vi "OCRListAvialableLangs_Training.vi"(8 "error in (no error)":errorcluster) -> (0 "error out":errorcluster, 3 "Langs":string[](array[string]))   [LabVIEW 2019]
panel:
  out "standard error":string
  out "standard output":string
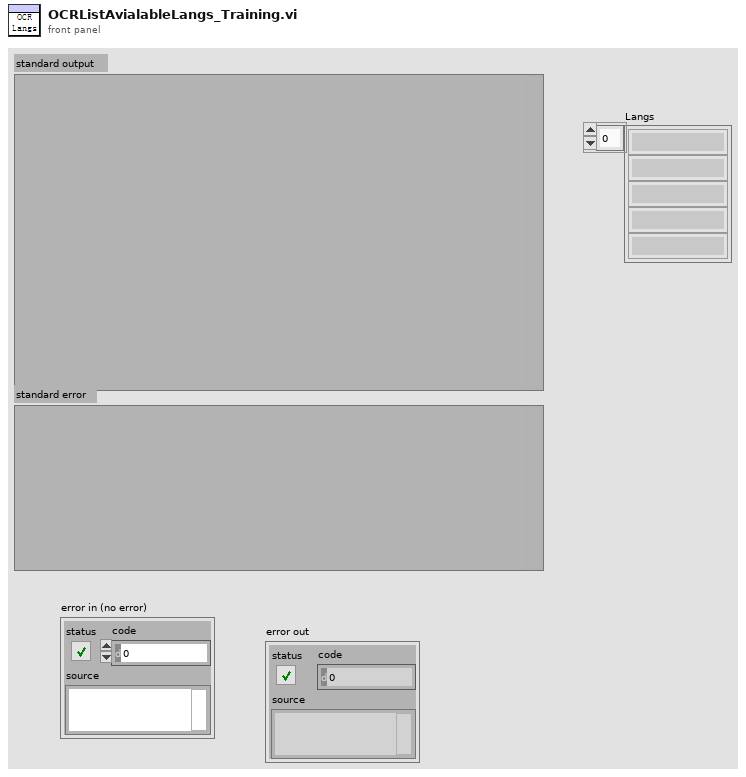
[diagram p1: front panel]
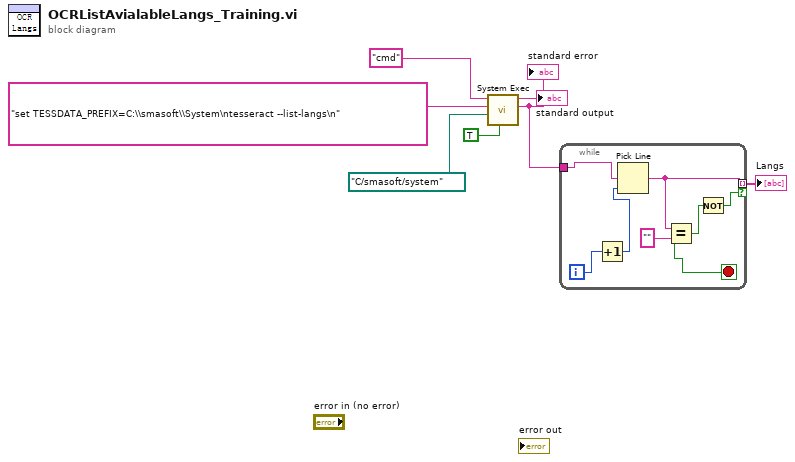
[diagram p0: block diagram]
diagram:
  n1 = call <vilib>:"System Exec.vi"("run minimized? (F)"=TRUE, "working directory"=path "C:/smasoft/system", "standard input"="set TESSDATA_PREFIX=C:\\smasoft\\System\ntesseract --list-langs\n", "command line"="cmd") -> ("standard error"=w2:string, "standard output"=→"standard output":string)  [unwired: 4 in, 2 out]
  "standard error" <- w2
  n2 = while {
    tunnel: w2 -> [w14]
    tunnel: [w11] -> w1 mode=indexing if=w8
    i -> [w13]
    stop <- w9 stop-if-true
    n3 = Increment(x=w13) -> (x+1=w12:i32)
    n4 = Pick Line(multi-line string=w14, line index=w12) -> (output string=w11:string)  [unwired: 1 in]
    n5 = Equal?(x=w11, y="") -> (x = y?=w9:bool)
    n6 = Not(x=w9) -> (.not. x?=w8:bool)
  }
  "Langs" <- w1
